vi "MD4Logger.Async.vi"(10 "Parameters":variant, 11 "Process":refnum<class "Process.lvclass">) -> ()   [LabVIEW 2019, in "MD4Logger Engine.lvlib"]
uses:
  MD4Logger Engine.lvlib
  <vilib>/NI/NIVS Inline Async API/_VS Inline Async API/Process/Process.lvclass
  Shared/Compiled.Settings.ctl
  <vilib>/NI/NIVS Inline Async API/_VS Inline Async API/Process/Process.lvclass/Process.ctl
  <vilib>/NI/NIVS Inline Async API/_Data Access Engine/Access Type Classes/Read/Read.lvclass/Read.ctl
  <vilib>/NI/NIVS Inline Async API/_Data Access Engine/Data Access Engine/Methods/Read.Data.vi
  <vilib>/NI/NIVS Inline Async API/_VS Inline Async API/Process/Data Member Access/Read Data Access.vi
  <vilib>/NI/NIVS Inline Async API/_VS Inline Async API/Error Handling Process/SubVIs/Error.ConvertArray.vi
  <vilib>/NI/NIVS Inline Async API/_Data Access Engine/Access Type Classes/Read/Read.ProcessData.vi
  Shared/Constants.vi
  <vilib>/NI/NIVS Inline Async API/_Data Access Engine/Data Access Engine/Methods/Read.Lookup.vi
  <vilib>/NI/NIVS Inline Async API/_Data Access Engine/Data Access Engine/Data Access Engine.lvclass
  Shared/MD4Logger Shared.lvlib
  <vilib>/NI VeriStand/Custom Device Tools/Custom Device Utility Library/Custom Device Utility Library.lvlib
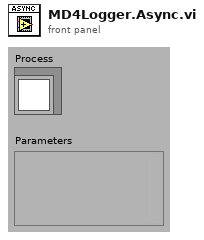
[diagram p1: front panel]
types:
  T1 = typedef "MD4Logger Shared.lvlib/Compiled.Settings.ctl" = cluster{"Name":string, "Folder Path":path, "Channnel Names":cluster{"Name":string, "Unit":string}[], "File Name":string}
  T2 = typedef "Data Access Engine.lvlib/Data Access Engine.lvclass/Read.DVR.ctl" = refnum<data-value>
  T3 = cluster{"MDF4 File Reference out":i64, "Channels Count":i32, "Stream Reference out":i64, "CreateFile Command Val":dbl, "error IO":errorcluster}
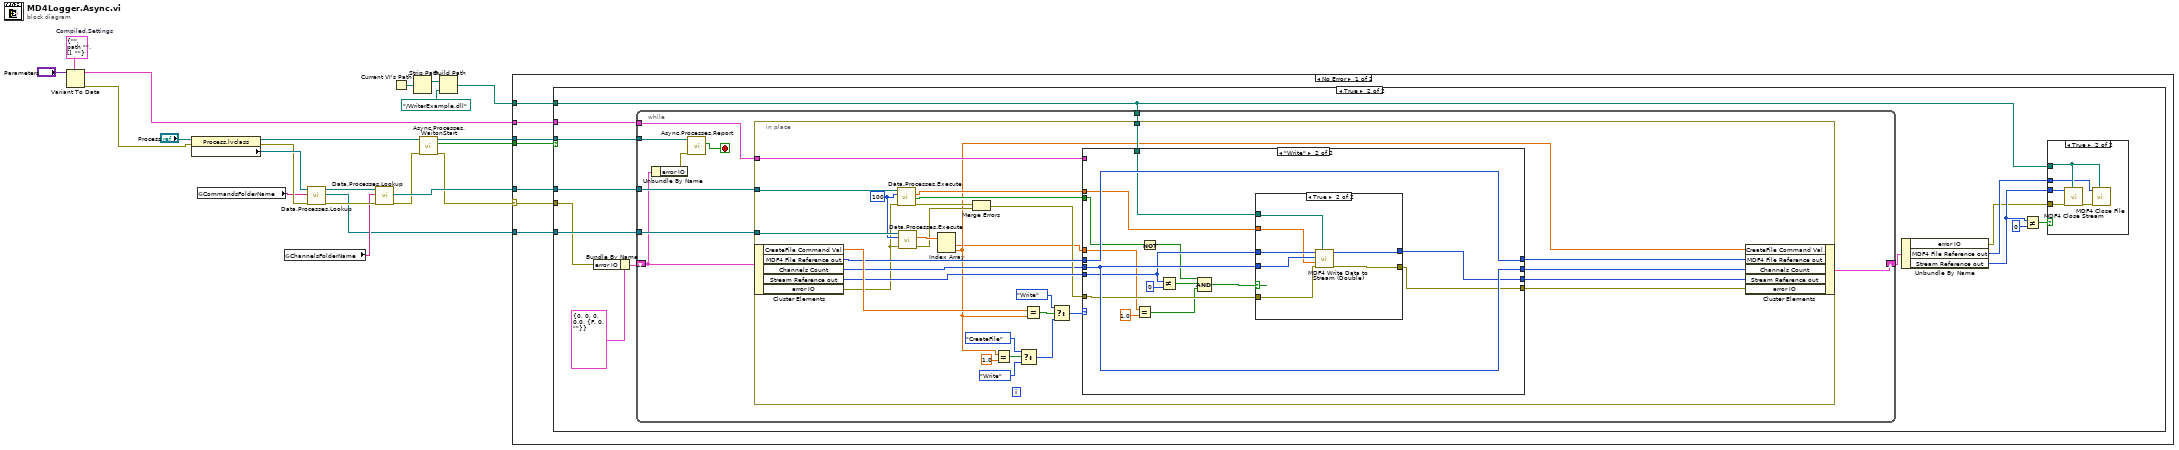
[diagram p0: block diagram]
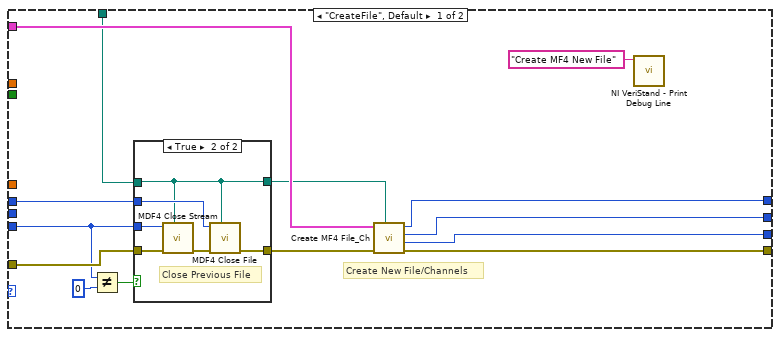
[diagram p4: hidden frame]
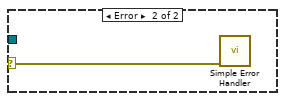
[diagram p7: hidden frame]
diagram:
  w11 = T1 {"Name"="", "Folder Path"=path "", "Channnel Names"=[], "File Name"=""}  # Compiled.Settings
  n1 = Variant To Data(type=w11, Variant="Parameters") -> (data=w4:T1, error out=w8:errorcluster)  [unwired: 1 in]
  n2 = property class="Process.lvclass"(reference="Process", error in=w8) -> (reference out=w15:refnum<class "Process.lvclass">, error out=w13:errorcluster, "Data Member Access:Data Access"=w14:refnum<class "Data Access Engine.lvclass">)
  n3 = global read "Constants.vi" "CommandsFolderName"() -> (w6:string)
  n4 = global read "Constants.vi" "ChannelsFolderName"() -> (w10:string)
  n5 = call-poly <vilib>:"Data.Processes.Lookup.vi"("error in (no error)"=w13, "Name"=w6, "Data Access API in"=w14) -> ("error out"=w19:errorcluster, "Ref"=w5:T2, "Data Access API out"=w18:refnum<class "Data Access Engine.lvclass">)  [unwired: 5 in, 1 out]
  n6 = call-poly <vilib>:"Data.Processes.Lookup.vi"("error in (no error)"=w19, "Name"=w10, "Data Access API in"=w18) -> ("error out"=w17:errorcluster, "Ref"=w20:T2)  [unwired: 5 in, 2 out]
  n7 = Current VI's Path() -> (path=w2:path)
  n8 = Strip Path(path=w2) -> (stripped path=w3:path)  [unwired: 1 out]
  n9 = call <vilib>:"Async.Processes.WaitonStart.vi"("error in (no error)"=w17, "Process"=w15) -> ("error out"=w9:errorcluster, "Execute"=w22:bool, "Process out"=w21:refnum<class "Process.lvclass">)  [unwired: 7 in]
  n10 = Build Path(base path=w3, name or relative path=path "../WriterExample.dll") -> (appended path=w7:path)
  n11 = case shown="No Error" w9 {
    selector: w9 -> [w26 w135]
    tunnel: w22 -> [w29 _]
    tunnel: w21 -> [w28 _]
    tunnel: w20 -> [w27 _]
    tunnel: w7 -> [w25 _]
    tunnel: w5 -> [w24 _]
    tunnel: w4 -> [w23 _]
    frame No Error {
      n12 = case shown="True" w29 {
        tunnel: w26 -> [_ w31]
        tunnel: w28 -> [_ w42]
        tunnel: w27 -> [_ w43]
        tunnel: w25 -> [_ w35]
        tunnel: w24 -> [_ w41]
        tunnel: w23 -> [_ w40]
        frame False {
        }
        frame True {
          n13 = Bundle By Name(cluster=T3 {"MDF4 File Reference out"=0, "Channels Count"=0, "Stream Reference out"=0, "CreateFile Command Val"=0.0, "error IO"={"status"=FALSE, "code"=0, "source"=""}}, "error IO"=w31) -> (w32:T3)
          n14 = while {
            tunnel: w42 -> [w49]
            tunnel: w43 -> [w57]
            tunnel: w41 -> [w56]
            shift-right: [w53] -> w37
            shift-left: w32 -> [w51]
            tunnel: w35 -> [w55]
            tunnel: w40 -> [w54]
            stop <- w52 stop-if-true
            n15 = Unbundle By Name(w51) -> ("error IO"=w50:errorcluster)
            n16 = call <vilib>:"Async.Processes.Report.vi"("Error"=w50, "Process in"=w49) -> ("Stop"=w52:bool)  [unwired: 8 in, 1 out]
            n17 = in-place {
              in-place-border: w57 -> [w87]
              in-place-border: w56 -> [w86]
              in-place-border: w55 -> [w73]
              in-place-border: w54 -> [w68]
              w69 = 100 ("timeout ms")
              n18 = in-place-cluster #1(w51) -> ("CreateFile Command Val"=w77:dbl, "MDF4 File Reference out"=w75:i64, "Channels Count"=w64:i32, "Stream Reference out"=w74:i64, "error IO"=w60:errorcluster)
              n19 = call-poly <vilib>:"Data.Processes.Execute.vi"("error in (no error)"=w60, "timeout ms"=w69, "Ref"=w87) -> ("error out"=w72:errorcluster, "Timeout?"=w63:bool, "Values"=w62:dbl[])  [unwired: 6 in]
              n20 = call-poly <vilib>:"Data.Processes.Execute.vi"("error in (no error)"=w60, "timeout ms"=w69, "Ref"=w86) -> ("error out"=w70:errorcluster, "Values"=w85:dbl[])  [unwired: 6 in, 1 out]
              n21 = Index Array(array=w85) -> (element #1=w58:dbl, element #2=w59:dbl)  [unwired: 2 in]
              n22 = Merge Errors(w72, w70) -> (w71:errorcluster)
              n23 = Equal?(x=w59, y=1.0) -> (x = y?=w81:bool)
              n24 = Select(t=enum16{"CreateFile", "Write"}."CreateFile", s=w81, f=enum16{"CreateFile", "Write"}."Write") -> (s? t:f=w78:enum16{"CreateFile", "Write"})
              n25 = Equal?(x=w77, y=w59) -> (x = y?=w84:bool)
              n26 = Select(t=enum16{"CreateFile", "Write"}."Write", s=w84, f=w78) -> (s? t:f=w76:enum16{"CreateFile", "Write"})
              n27 = case shown="\"Write\"" w76 {
                tunnel: w75 -> [w101 w125]
                tunnel: w74 -> [w99 w117]
                tunnel: w73 -> [w90 w116]
                tunnel: w71 -> [w100 w119]
                tunnel: w68 -> [w96 _]
                tunnel: [w94 w125] -> w67
                tunnel: [w93 w122] -> w66
                tunnel: [w92 w118] -> w65
                tunnel: w64 -> [_ w122]
                tunnel: w63 -> [_ w123]
                tunnel: w62 -> [_ w121]
                tunnel: [w91 w120] -> w61
                tunnel: w58 -> [_ w115]
                frame "CreateFile", Default {
                  # "Create New File/Channels"
                  n28 = Not Equal?(x=w99, y=i64 0) -> (x != y?=w97:bool)
                  n29 = case shown="True" w97 {
                    tunnel: w101 -> [_ w109]
                    tunnel: w90 -> [w102 w104]
                    tunnel: w100 -> [w103 w107]
                    tunnel: w99 -> [_ w106]
                    tunnel: [w103 w105] -> w95
                    tunnel: [w102 w104] -> w88
                    frame False {
                    }
                    frame True {
                      # "Close Previous File"
                      n30 = call "MDF4 Close Stream.vi"("path in"=w104, "Error In"=w107, "Stream Reference in"=w106) -> ("Error Out"=w108:errorcluster)  [unwired: 7 in, 1 out]
                      n31 = call "MDF4 Close File.vi"("path in"=w104, "Error In"=w108, "MDF4 File Reference in"=w109) -> ("Error Out"=w105:errorcluster)  [unwired: 7 in, 1 out]
                    }
                  }
                  n32 = call "Create MF4 File_Ch.vi"("DLL path"=w88, "Error In"=w95, "input cluster"=w96) -> ("Error Out"=w91:errorcluster, "Stream Reference out"=w92:i64, "Channels Count"=w93:i32, "MDF4 File Reference out"=w94:i64)  [unwired: 5 in]
                  n33 = call <vilib>:"NI VeriStand - Print Debug Line.vi"("Message"="Create MF4 New File") -> ()  [unwired: 10 in, 1 out]
                }
                frame "Write" {
                  n34 = Equal?(x=w115, y=1.0) -> (x = y?=w111:bool)
                  n35 = Not(x=w123) -> (.not. x?=w113:bool)
                  n36 = Not Equal?(x=w117, y=i64 0) -> (x != y?=w112:bool)
                  n37 = Compound Arithmetic op=AND(w113, w112, w111) -> (w110:bool)
                  n38 = case shown="True" w110 {
                    tunnel: [w126 w130] -> w120
                    tunnel: [w127 w134] -> w118
                    tunnel: w117 -> [w127 w133]
                    tunnel: w122 -> [_ w132]
                    tunnel: w121 -> [_ w131]
                    tunnel: w119 -> [w126 w129]
                    tunnel: w116 -> [_ w128]
                    frame False {
                    }
                    frame True {
                      n39 = call "MDF4 Write Data to Stream (Double).vi"("path in"=w128, "Error In"=w129, "data"=w131, "chan_count"=w132, "Stream Reference in"=w133) -> ("Error Out"=w130:errorcluster, "Stream Reference out"=w134:i64)  [unwired: 5 in]
                    }
                  }
                }
              }
              n40 = in-place-cluster #1("CreateFile Command Val"=w59, "MDF4 File Reference out"=w67, "Channels Count"=w66, "Stream Reference out"=w65, "error IO"=w61) -> (w53:T3)
            }
          }
          n41 = Unbundle By Name(w37) -> ("error IO"=w30:errorcluster, "MDF4 File Reference out"=w36:i64, "Stream Reference out"=w34:i64)
          n42 = Not Equal?(x=w34, y=i64 0) -> (x != y?=w39:bool)
          n43 = case shown="True" w39 {
            tunnel: w36 -> [_ w44]
            tunnel: w35 -> [_ w47]
            tunnel: w30 -> [_ w46]
            tunnel: w34 -> [_ w45]
            frame False {
            }
            frame True {
              n44 = call "MDF4 Close Stream.vi"("path in"=w47, "Error In"=w46, "Stream Reference in"=w45) -> ("Error Out"=w48:errorcluster)  [unwired: 7 in, 1 out]
              n45 = call "MDF4 Close File.vi"("path in"=w47, "Error In"=w48, "MDF4 File Reference in"=w44) -> ()  [unwired: 7 in, 2 out]
            }
          }
        }
      }
    }
    frame Error {
      n46 = call <vilib>:"Simple Error Handler.vi"("error in (no error)"=w135) -> ()  [unwired: 4 in, 5 out]
    }
  }
